vi "WSVCAP SHL Host LL RFFE Convert Bit Array to Channel Bytes.vi"(0 "Bit Array":u64[](array[numeric]) format="%016b") -> (4 "RFFE Read Data [Socket Ordered]":u8[][](array[numeric]) format="%.0x")   [LabVIEW 2012]
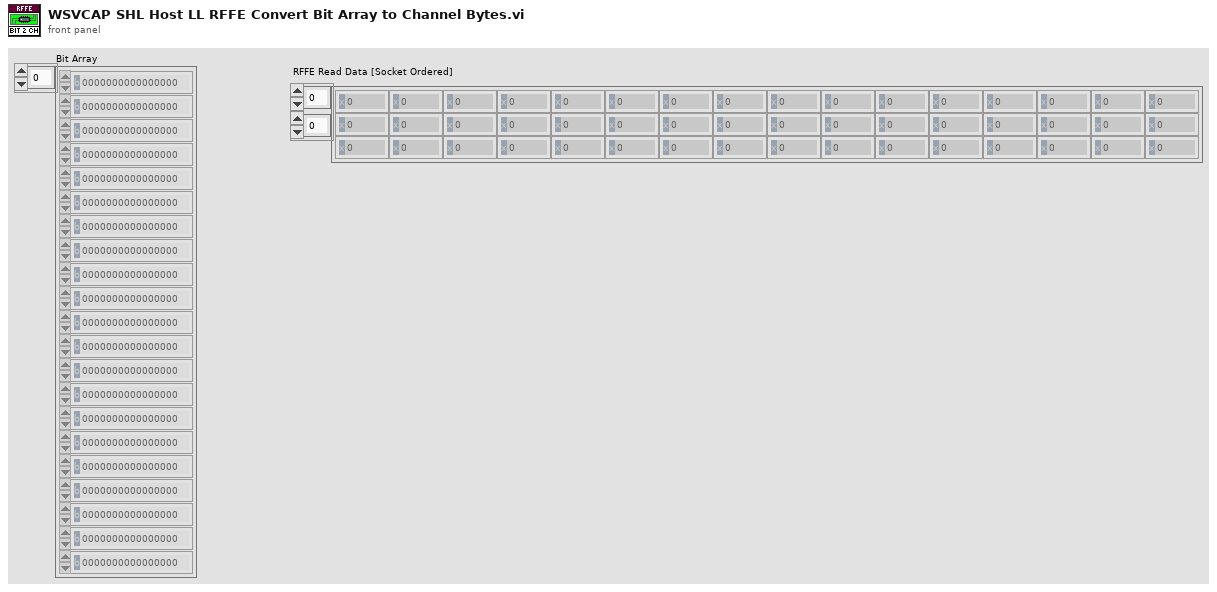
[diagram p1: front panel]
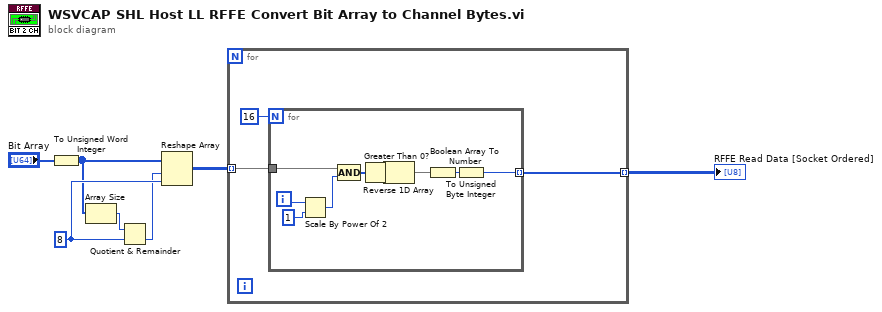
[diagram p0: block diagram]
diagram:
  w4 = 8 ("Read Data In")
  n1 = To Unsigned Word Integer(number="Bit Array") -> (unsigned 16bit integer=w1:u16[])
  n2 = Array Size(array=w1) -> (size(s)=w6:i32)
  n3 = Quotient & Remainder(x=w6, y=w4) -> (floor(x/y)=w3:i32)  [unwired: 1 out]
  n4 = Reshape Array(w1, w3, w4) -> (w5:u16[][])
  n5 = for {
    tunnel: w5 -> [w10] mode=indexing
    tunnel: [w8] -> w2 mode=indexing
    n6 = for {
      N: 16 -> [_]
      tunnel: w10 -> [w18]
      tunnel: [w14] -> w8 mode=indexing
      i -> [w13]
      n7 = Scale By Power Of 2(n=w13, x=u16 1) -> (x*2^n=w17:u16)
      n8 = Compound Arithmetic op=AND(w18, w17) -> (w16:u16[])
      n9 = Greater Than 0?(x=w16) -> (x > 0?=w12:bool[])
      n10 = Reverse 1D Array(array=w12) -> (reversed array=w11:bool[])
      n11 = Boolean Array To Number(Boolean array=w11) -> (number=w15:u32)
      n12 = To Unsigned Byte Integer(number=w15) -> (unsigned 8bit integer=w14:u8)
    }
  }
  "RFFE Read Data [Socket Ordered]" <- w2
